vi "WriteLog.vi"(8 "error in (no error)":errorcluster, 11 "Log in":refnum<class "Log.lvclass">) -> (0 "error out":errorcluster, 3 "Log out":refnum<class "Log.lvclass">)   [LabVIEW 2018, in "Log.lvclass"]
uses:
  Log.lvclass
  Log.lvclass/Log.ctl
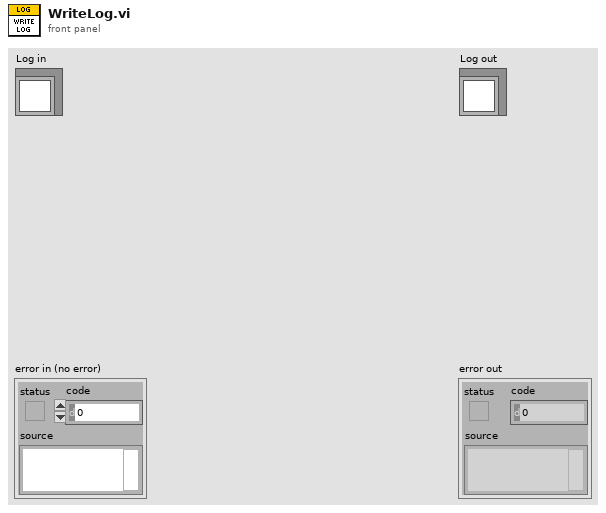
[diagram p1: front panel]
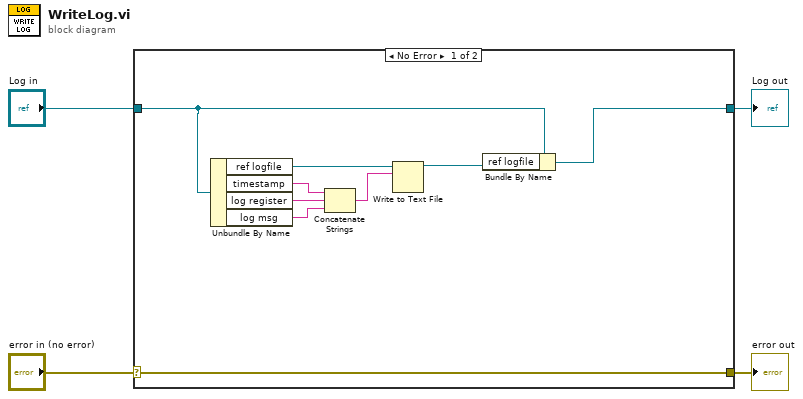
[diagram p0: block diagram]
diagram:
  n1 = case shown="No Error" "error in (no error)" {
    selector: "error in (no error)" -> [w13 w15]
    tunnel: [w13 w15] -> w3
    tunnel: [w11 w14] -> w1
    tunnel: "Log in" -> [w12 w14]
    frame No Error {
      n2 = Unbundle By Name(w12) -> ("ref logfile"=w10:refnum<file>, "timestamp"=w8:string, "log register"=w7:string, "log msg"=w6:string)
      n3 = Concatenate Strings(w8, w7, w6) -> (w5:string)
      n4 = Write to Text File(file (use dialog)=w10, text=w5) -> (refnum out=w9:refnum<file>)  [unwired: 2 in, 2 out]
      n5 = Bundle By Name(cluster=w12, "ref logfile"=w9) -> (w11:refnum<class "Log.lvclass">)
    }
    frame Error {
    }
  }
  "error out" <- w3
  "Log out" <- w1
